vi "Write CmdSocket.vi"(8 "error in (no error)":errorcluster, 10 "CmdSocket":refnum<class "Socket.Base.lvclass">, 11 "C37.118 PMU in":refnum<class "C37.118 PMU.lvclass">) -> (0 "error out":errorcluster, 3 "C37.118 PMU out":refnum<class "C37.118 PMU.lvclass">)   [LabVIEW 2014, in "SensorPlugins.lvlib" / "C37.118 PMU.lvclass"]
uses:
  C37.118 PMU.lvclass
  <userlib>/NIST/Socket Class/Classes/Socket.Base/Socket.Base.lvclass
  C37.118 PMU.lvclass/C37.118 PMU.ctl
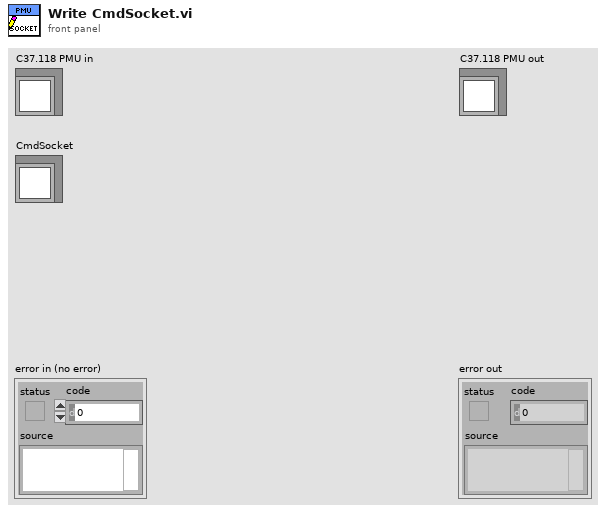
[diagram p1: front panel]
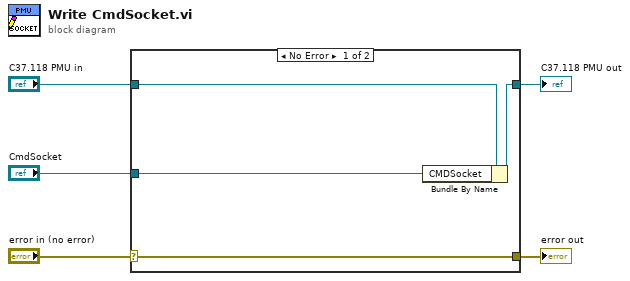
[diagram p0: block diagram]
diagram:
  n1 = case shown="No Error" "error in (no error)" {
    selector: "error in (no error)" -> [w9 w10]
    tunnel: [w9 w10] -> w4
    tunnel: [w7 w11] -> w2
    tunnel: "C37.118 PMU in" -> [w8 w11]
    tunnel: "CmdSocket" -> [w6 _]
    frame No Error {
      n2 = Bundle By Name(cluster=w8, "CMDSocket"=w6) -> (w7:refnum<class "C37.118 PMU.lvclass">)
    }
    frame Error {
    }
  }
  "error out" <- w4
  "C37.118 PMU out" <- w2
